vi "niRFUtil WFM Subtract Waveforms (complex wfm).vi"(2 "Waveform 2 In":T1 {"y" format="%.2f"; "dx" format="%^.2e"; "x0" format="%^.2e"}, 3 "Waveform 1 In":T1 {"y" format="%.2f"; "dx" format="%^.2e"; "x0" format="%^.2e"}) -> (1 "Waveform 1 - Waveform 2":T1 {"y" format="%.2f"; "dx" format="%^.2e"; "x0" format="%^.2e"})   [LabVIEW 2015, in "niRFUtil.lvlib"]
doc: "(c) Copyright 2006, National Instruments, Inc. This VI may not be duplicated, sold, or distributed without written consent from National Instruments."
uses:
  niRFUtil.lvlib
  Includes/niRFUtil INC Complex Waveform.ctl
  Includes/niRFUtil INC Complex Array.ctl
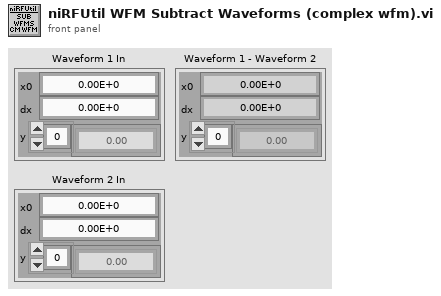
[diagram p1: front panel]
types:
  T1 = typedef "niRFUtil.lvlib/niRFUtil INC Complex Waveform.ctl" = cluster{"x0":dbl, "dx":dbl, "y":T2}
  T2 = typedef "niRFUtil.lvlib/niRFUtil INC Complex Array.ctl" = csg[]
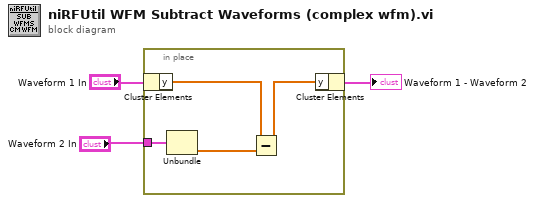
[diagram p0: block diagram]
diagram:
  n1 = in-place {
    in-place-border: "Waveform 2 In" -> [w7]
    n2 = in-place-cluster #1("Waveform 1 In") -> ("y"=w5:T2)
    n3 = Unbundle(w7) -> ("y"=w6:T2)  [unwired: 2 out]
    n4 = Subtract(x=w5, y=w6) -> (x-y=w4:T2)
    n5 = in-place-cluster #1("y"=w4) -> (→"Waveform 1 - Waveform 2":T1)
  }
